vi "Delete values below threshold from array.vi"(9 "Threshold":i32=100, 11 "Values":i32[](array[numeric])) -> (3 "Values out":i32[](array[numeric]))   [LabVIEW 2017]
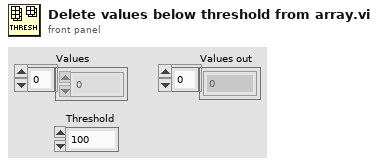
[diagram p1: front panel]
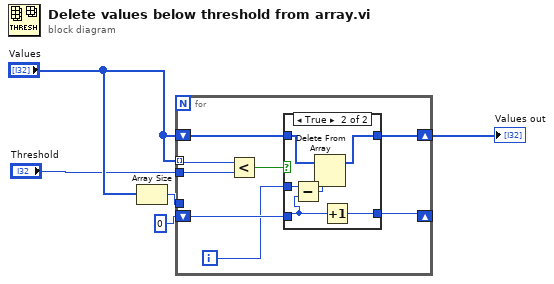
[diagram p0: block diagram]
diagram:
  n1 = Array Size(array="Values") -> (size(s)=w4:i32)
  n2 = for {
    tunnel: "Values" -> [w12] mode=indexing
    shift-right: [w10] -> w2
    shift-left: "Values" -> [w11]
    tunnel: w4 -> [_]
    shift-right: [w8] -> _
    shift-left: 0 -> [w9]
    tunnel: "Threshold" -> [w6]
    i -> [w7]
    n3 = Less?(x=w12, y=w6) -> (x < y?=w13:bool)
    n4 = case shown="True" w13 {
      tunnel: w11 -> [w15 w21]
      tunnel: [w15 w20] -> w10
      tunnel: w9 -> [w14 w17]
      tunnel: [w14 w19] -> w8
      tunnel: w7 -> [_ w18]
      frame False {
      }
      frame True {
        n5 = Subtract(x=w18, y=w17) -> (x-y=w16:i32)
        n6 = Delete From Array(array=w21, index=w16) -> (array with subset deleted=w20:i32[])  [unwired: 1 in, 1 out]
        n7 = Increment(x=w17) -> (x+1=w19:i32)
      }
    }
  }
  "Values out" <- w2
